vi "Write Current Logic Outputs.vi"(10 "Current Logic Outputs":bool[](array[boolean]), 11 "LogicIO in":refnum<class "LogicIO.lvclass">) -> (3 "LogicIO out":refnum<class "LogicIO.lvclass">)   [LabVIEW 2016, in "Hardware.lvlib" / "LogicIO.lvlib" / "LogicIO.lvclass"]
uses:
  <userlib>/Common Components/Hardware/LogicIO/LogicIO/LogicIO.lvclass
  <userlib>/Common Components/Hardware/LogicIO/LogicIO/LogicIO.lvclass/LogicIO.ctl
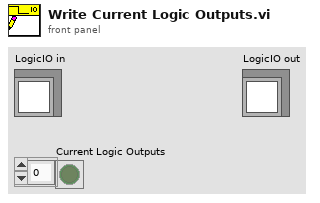
[diagram p1: front panel]
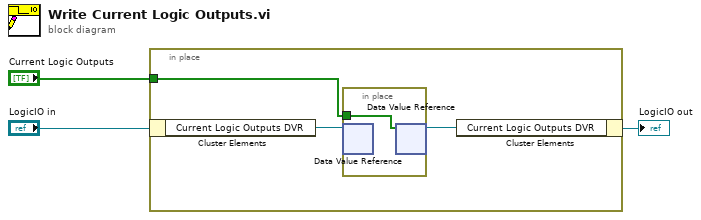
[diagram p0: block diagram]
diagram:
  n1 = in-place {
    in-place-border: "Current Logic Outputs" -> [w6]
    n2 = in-place-cluster #1("LogicIO in") -> ("Current Logic Outputs DVR"=w5:refnum<data-value>)
    n3 = in-place {
      in-place-border: w6 -> [w7]
      n4 = in-place-dvr #2(w5) -> ()  [unwired: 2 out]
      n5 = in-place-dvr #2(w7) -> (w4:refnum<data-value>)  [unwired: 1 out]
    }
    n6 = in-place-cluster #1("Current Logic Outputs DVR"=w4) -> (→"LogicIO out":refnum<class "LogicIO.lvclass">)
  }
